vi "Write Update Channel OOB.vi"(8 "error in (no error)":errorcluster, 10 "Update OOB":bool, 11 "CIFCorePlugin in":refnum<class "CIFCorePlugin.lvclass">) -> (0 "error out":errorcluster, 3 "CIFCorePlugin out":refnum<class "CIFCorePlugin.lvclass">)   [LabVIEW 2021, in "CIFCorePlugin.lvclass"]
uses:
  CIFCorePlugin.lvclass
  CIFCorePlugin.lvclass/CIFCorePlugin.ctl
  Channels/CIFChannelMng/CIFChannelMng.lvclass/CIFChannelMng.ctl
  Channels/CIFChannelMng/CIFChannelMng.lvclass
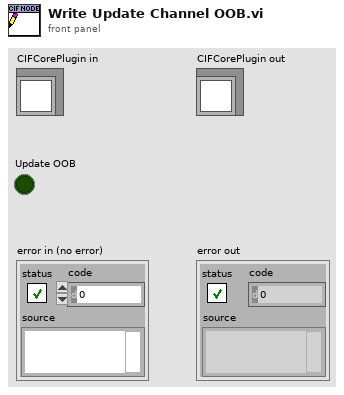
[diagram p1: front panel]
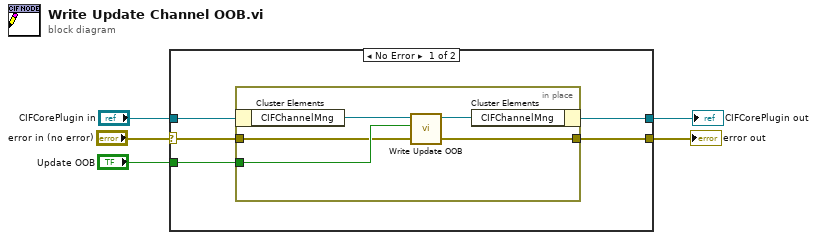
[diagram p0: block diagram]
diagram:
  n1 = case shown="No Error" "error in (no error)" {
    selector: "error in (no error)" -> [w8 w16]
    tunnel: [w7 w16] -> w4
    tunnel: [w6 w17] -> w2
    tunnel: "CIFCorePlugin in" -> [w9 w17]
    tunnel: "Update OOB" -> [w10 _]
    frame No Error {
      n2 = in-place {
        in-place-border: w10 -> [w15]
        in-place-border: w8 -> [w12]
        in-place-border: [w11] -> w7
        n3 = in-place-cluster #1(w9) -> ("CIFChannelMng"=w14:refnum<class "CIFChannelMng.lvclass">)
        n4 = call "Write Update OOB.vi"("error in (no error)"=w12, "Update OOB"=w15, "CIFChannelMng in"=w14) -> ("error out"=w11:errorcluster, "CIFChannelMng out"=w13:refnum<class "CIFChannelMng.lvclass">)  [unwired: 7 in]
        n5 = in-place-cluster #1("CIFChannelMng"=w13) -> (w6:refnum<class "CIFCorePlugin.lvclass">)
      }
    }
    frame Error {
    }
  }
  "error out" <- w4
  "CIFCorePlugin out" <- w2
